vi "FPGA_controller.vi"() -> ()   [LabVIEW 2017]
uses:
  <vilib>/rvi/Emulation/niFpgaGetClockAttributes.vi
  <vilib>/rvi/Emulation/niFpgaSctlEmulationGetInTimedLoop.vi
  <vilib>/rvi/Emulation/niFpgaEmulationReportErrorSimple.vi
  <vilib>/rvi/eio/common/nirviEmuTemplateMethod_errors.vi
  <vilib>/rvi/Emulation/niFpgaCriticalErrorInLSC.vi
  <vilib>/eio/EIONode/EIONode.xnode
panel:
  out "VALID":bool
  in  "Scale x2":fxp<+/-,32,16>=10.0 format="%#_21g"
  in  "m_first x2":fxp<+/-,49,33>=4.9499969482421875 format="%#_26g"
  in  "Offset x2":fxp<+/-,48,32> format="%#_26g"
  in  "1/eta x":fxp<+,8,8>=200.0 format="%#_21g"
  in  "m_first x1":fxp<+/-,49,33>=0.649993896484375 format="%#_26g"
  in  "Offset x1":fxp<+/-,48,32> format="%#_26g"
  in  "Scale x1":fxp<+/-,32,16>=5.0 format="%#_21g"
  in  "stop 2":bool
  # "STATES CONVERSION"
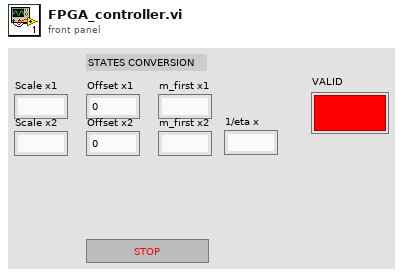
[diagram p1: front panel]
types:
  T1 = cluster{"Boolean array[0]":bool, "Boolean array[1]":bool, "Boolean array[2]":bool, "Boolean array[3]":bool, "Boolean array[4]":bool, "Boolean array[5]":bool, "Boolean array[6]":bool, "Boolean array[7]":bool, "Boolean array[8]":bool, "Boolean array[9]":bool, "Boolean array[10]":bool, "Boolean array[11]":bool, "Boolean array[12]":bool, "Boolean array[13]":bool, "Boolean array[14]":bool, "Boolean array[15]":bool}
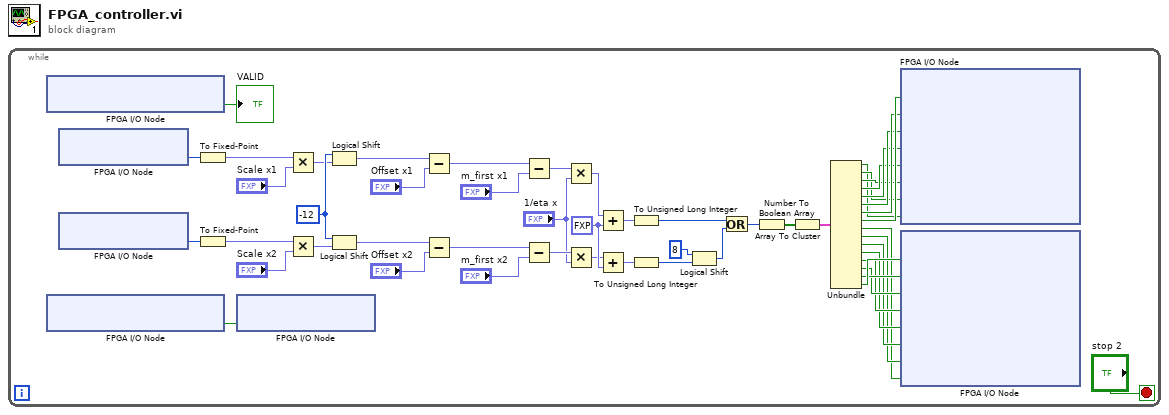
[diagram p0: block diagram]
diagram:
  n1 = while {
    stop <- "stop 2" stop-if-true
    w24 = fxp<+,2,1> 0.5 ("y")
    w22 = i16 -12 ("y")
    n2 = xnode "FPGA I/O Node"() -> ("Component-Level IP\\po1"=→"VALID":bool)  [unwired: 1 in, 1 out]
    n3 = xnode "FPGA I/O Node"() -> ("Component-Level IP\\po0"=w31:bool)  [unwired: 1 in, 1 out]
    n4 = xnode "FPGA I/O Node"() -> ("ConnectorA/AI0"=w51:u16)  [unwired: 1 in, 1 out]
    n5 = xnode "FPGA I/O Node"() -> ("ConnectorA/AI1"=w50:u16)  [unwired: 1 in, 1 out]
    n6 = To Fixed-Point(number=w51) -> (fixed-point=w3:fxp<+,16,16>)  [unwired: 1 in]
    n7 = To Fixed-Point(number=w50) -> (fixed-point=w2:fxp<+,16,16>)  [unwired: 1 in]
    n8 = xnode "FPGA I/O Node"("ConnectorA/DIO0"=w31) -> ()  [unwired: 1 in, 1 out]
    n9 = Multiply(x=w3, y="Scale x1") -> (x*y=w21:fxp<+/-,48,32>)
    n10 = Multiply(x=w2, y="Scale x2") -> (x*y=w25:fxp<+/-,48,32>)
    n11 = Logical Shift(y=w22, x=w21) -> (x << y=w18:fxp<+/-,48,32>)
    n12 = Logical Shift(y=w22, x=w25) -> (x << y=w16:fxp<+/-,48,32>)
    n13 = Subtract(x=w18, y="Offset x1") -> (x-y=w19:fxp<+/-,49,33>)
    n14 = Subtract(x=w16, y="Offset x2") -> (x-y=w17:fxp<+/-,49,33>)
    n15 = Subtract(x=w19, y="m_first x1") -> (x-y=w20:fxp<+/-,50,34>)
    n16 = Subtract(x=w17, y="m_first x2") -> (x-y=w15:fxp<+/-,50,34>)
    n17 = Multiply(x=w20, y="1/eta x") -> (x*y=w1:fxp<+/-,58,42>)
    n18 = Multiply(x=w15, y="1/eta x") -> (x*y=w14:fxp<+/-,58,42>)
    n19 = Add(x=w1, y=w24) -> (x+y=w30:fxp<+/-,58,42>)
    n20 = Add(x=w14, y=w24) -> (x+y=w23:fxp<+/-,58,42>)
    n21 = To Unsigned Long Integer(number=w30) -> (unsigned 32bit integer=w26:u32)
    n22 = To Unsigned Long Integer(number=w23) -> (unsigned 32bit integer=w28:u32)
    n23 = Logical Shift(y=8, x=w28) -> (x << y=w27:u32)
    n24 = Or(x=w26, y=w27) -> (x .or. y?=w11:u32)
    n25 = Number To Boolean Array(number=w11) -> (Boolean array=w12:bool[])
    n26 = Array To Cluster(array=w12) -> (cluster=w32:T1)
    n27 = Unbundle(w32) -> ("Boolean array[0]"=w33:bool, "Boolean array[1]"=w34:bool, "Boolean array[2]"=w35:bool, "Boolean array[3]"=w36:bool, "Boolean array[4]"=w37:bool, "Boolean array[5]"=w38:bool, "Boolean array[6]"=w39:bool, "Boolean array[7]"=w40:bool, "Boolean array[8]"=w41:bool, "Boolean array[9]"=w42:bool, "Boolean array[10]"=w43:bool, "Boolean array[11]"=w44:bool, "Boolean array[12]"=w45:bool, "Boolean array[13]"=w46:bool, "Boolean array[14]"=w47:bool, "Boolean array[15]"=w48:bool)
    n28 = xnode "FPGA I/O Node"("Component-Level IP\\pi00"=w40, "Component-Level IP\\pi01"=w39, "Component-Level IP\\pi02"=w38, "Component-Level IP\\pi03"=w37, "Component-Level IP\\pi04"=w36, "Component-Level IP\\pi05"=w35, "Component-Level IP\\pi06"=w34, "Component-Level IP\\pi07"=w33) -> ()  [unwired: 8 in, 8 out]
    n29 = xnode "FPGA I/O Node"("Component-Level IP\\pi08"=w48, "Component-Level IP\\pi09"=w47, "Component-Level IP\\pi10"=w46, "Component-Level IP\\pi11"=w45, "Component-Level IP\\pi12"=w44, "Component-Level IP\\pi13"=w43, "Component-Level IP\\pi14"=w42, "Component-Level IP\\pi15"=w41) -> ()  [unwired: 8 in, 8 out]
  }
